vi "OE2031&OE2041_DATA Transmit.vi"(0 "Input Data":u8[](array[numeric]), 1 "Remote Mode":u16(ring) items=["USB"=0, "Ethernet"=3]) -> (2 "Total Data Array":dbl[][](array[numeric]), 3 "Parameter Values":T2, 4 "Trig_Count":u8[](array[numeric]), 5 "PLL&Overload":T1)   [LabVIEW 2011]
panel:
  out "Group":u16
  out "X":dbl[](array[numeric])
  out "Y":dbl[](array[numeric])
  out "Frequency":dbl[](array[numeric])
  out "XNoise":dbl[](array[numeric])
  out "XD1":dbl[](array[numeric])
  out "YD1":dbl[](array[numeric])
  out "XD2":dbl[](array[numeric])
  out "YD2":dbl[](array[numeric])
  out "AUXADC1":dbl[](array[numeric])
  out "AUXADC2":dbl[](array[numeric])
  out "AUXADC3":dbl[](array[numeric])
  out "AUXADC4":dbl[](array[numeric])
  out "XD3":dbl[](array[numeric])
  out "YD3":dbl[](array[numeric])
  out "YNoise":dbl[](array[numeric])
  out "R":dbl[](array[numeric])
  out "Xita":dbl[](array[numeric])
  out "RD1":dbl[](array[numeric])
  out "XitaD1":dbl[](array[numeric])
  out "RD2":dbl[](array[numeric])
  out "XitaD2":dbl[](array[numeric])
  out "RD3":dbl[](array[numeric])
  out "XitaD3":dbl[](array[numeric])
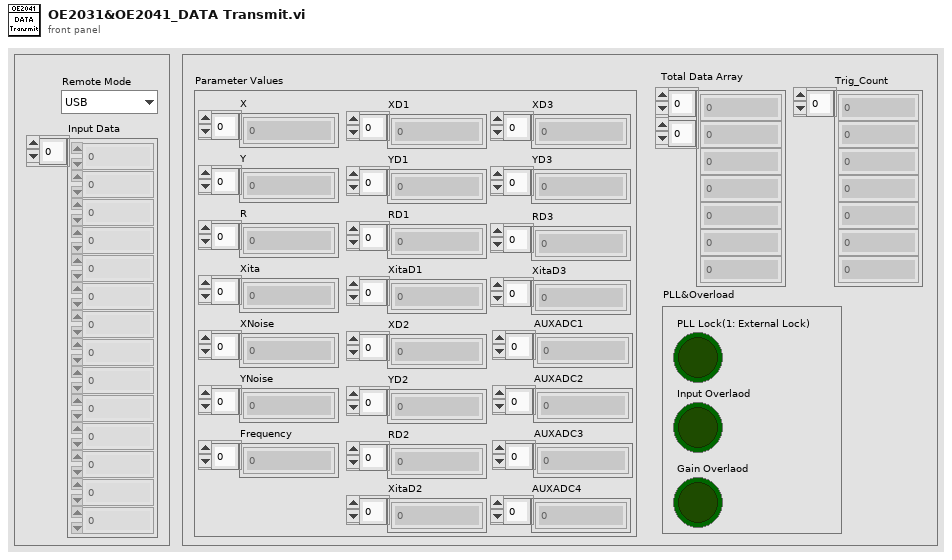
[diagram p1: front panel]
types:
  T1 = cluster{"PLL Lock(1: External Lock)":bool, "Input Overlaod":bool, "Gain Overlaod":bool}
  T2 = cluster{"X":dbl[], "Y":dbl[], "R":dbl[], "Xita":dbl[], "XNoise":dbl[], "YNoise":dbl[], "Frequency":dbl[], "XD1":dbl[], "YD1":dbl[], "RD1":dbl[], "XitaD1":dbl[], "XD2":dbl[], "YD2":dbl[], "RD2":dbl[], "XitaD2":dbl[], "XD3":dbl[], "YD3":dbl[], "RD3":dbl[], "XitaD3":dbl[], "AUXADC1":dbl[], "AUXADC2":dbl[], "AUXADC3":dbl[], "AUXADC4":dbl[]}
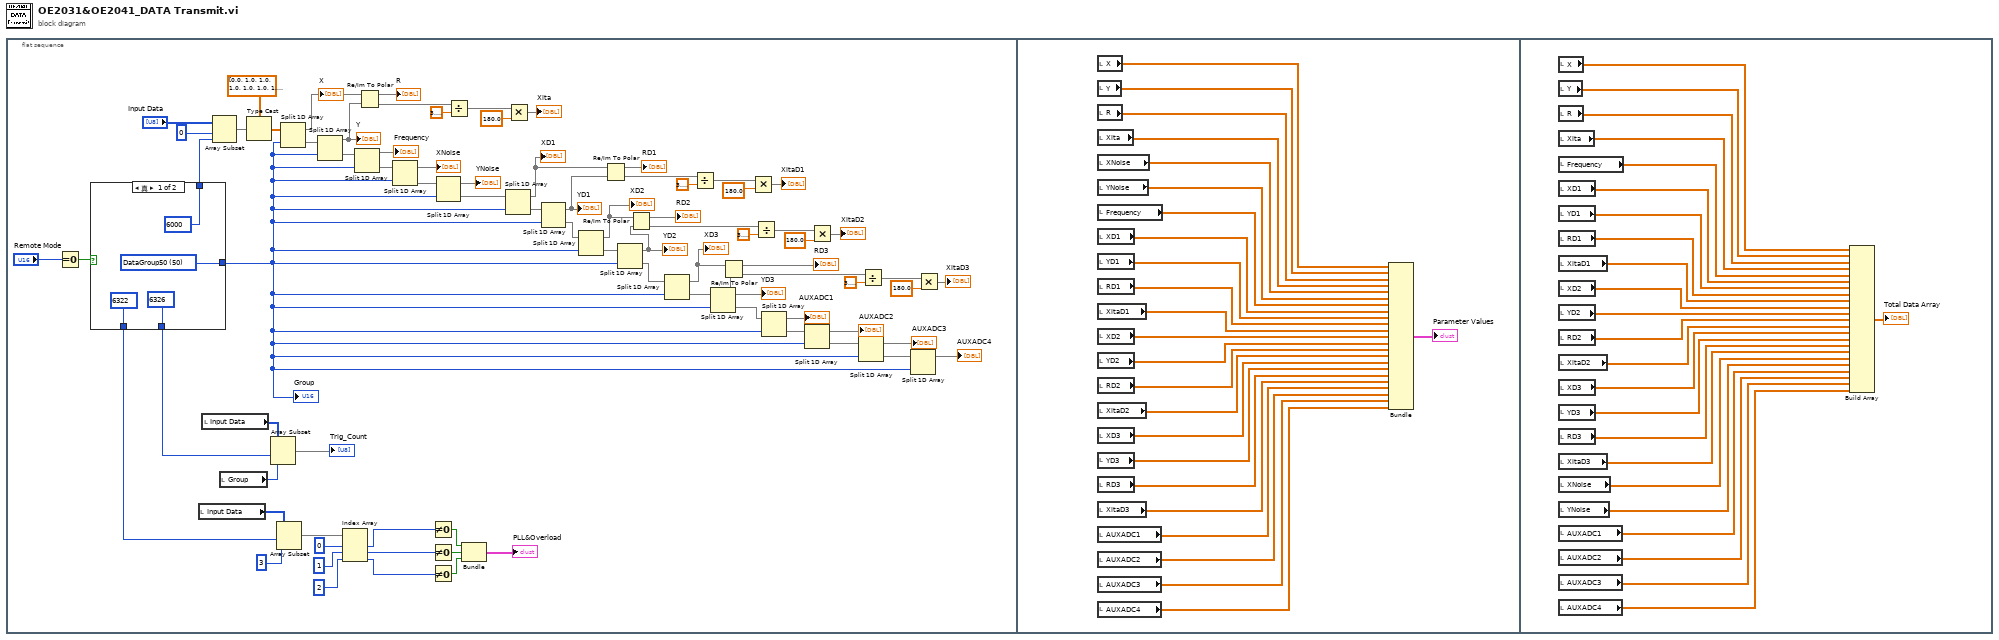
[diagram p0: block diagram]
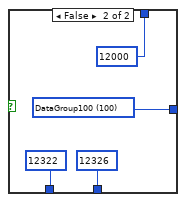
[diagram p2: hidden frame]
diagram:
  n1 = flat-sequence {
    frame #0 {
      n2 = Equal To 0?(x="Remote Mode") -> (x = 0?=w18:bool)
      n3 = case shown="真" w18 {
        tunnel: [w84 w88] -> w20
        tunnel: [6000 ("长度") 12000 ("长度")] -> w23
        tunnel: [6326 ("索引") 12326 ("索引")] -> w16
        tunnel: [6322 ("索引") 12322 ("索引")] -> w1
        frame True {
          w84 = u16 50 items=["unsignedInt8"=1, "unsignedInt16"=2, "unsignedInt32"=4, "unsignedInt64"=8, "Float"=80, "Double"=160, "StartLength"=2240, "DataGroup50"=50, "DataGroup100"=100, "DataGroup20"=20] ("数据类型")
        }
        frame False {
          w88 = u16 100 items=["unsignedInt8"=1, "unsignedInt16"=2, "unsignedInt32"=4, "unsignedInt64"=8, "Float"=80, "Double"=160, "StartLength"=2240, "DataGroup50"=50, "DataGroup100"=100, "DataGroup20"=20] ("数据类型")
        }
      }
      "Group" <- w20
      n4 = local read "Input Data"() -> (w14:u8[])
      n5 = local read "Input Data"() -> (w22:u8[])
      n6 = Array Subset(array="Input Data", index=0 ("索引"), length=w23) -> (w77:u8[])
      n7 = local read "Group"() -> (w19:u16)
      n8 = Type Cast(type=dbl[] [0.0, 1.0, 1.0, 1.0, 1.0, 1.0, 1.0, 1.0, 1.0, 1.0, 1.0, 1.0, 1.0, 1.0, 1.0, 1.0, 1.0, 1.0, 1.0, 1.0, 1.0, 1.0, 1.0, 1.0, 1.0, 1.0, 1.0, 1.0, 1.0, 1.0, 1.0, 1.0, 1.0, 1.0, 1.0, 1.0, 1.0, 1.0, 1.0, 1.0, 1.0, 1.0, 1.0, 1.0, 1.0, 1.0, 1.0, 1.0, 1.0, 1.0, 1.0, 1.0, 1.0, 1.0, 1.0, 1.0, 1.0, 1.0, 1.0, 1.0, 1.0, 1.0, 1.0, 1.0, 1.0, 1.0, 1.0, 1.0, 1.0, 1.0, 1.0, 1.0, 1.0, 1.0, 1.0, 1.0, 1.0, 1.0, 1.0, 1.0, 1.0, 1.0, 1.0, 1.0, 1.0, 1.0, 1.0, 1.0, 1.0, 1.0, 1.0, 1.0, 1.0, 1.0, 1.0, 1.0, 1.0, 1.0, 1.0, 1.0, 1.0, 1.0, 1.0, 1.0, 1.0, 1.0, 1.0, 1.0, 1.0, 1.0, 1.0, 1.0, 1.0, 1.0, 1.0, 1.0, 1.0, 1.0, 1.0, 1.0, 1.0, 1.0, 1.0, 1.0, 1.0, 1.0, 1.0, 1.0, 1.0, 1.0, 1.0, 1.0, 1.0, 1.0, 1.0, 1.0, 1.0, 1.0, 1.0, 1.0, 1.0, 1.0, 1.0, 1.0, 1.0, 1.0, 1.0, 1.0, 1.0, 1.0, 1.0, 1.0, 1.0, 1.0, 1.0, 1.0, 1.0, 1.0, 1.0, 1.0, 1.0, 1.0, 1.0, 1.0, 1.0, 1.0, 1.0, 1.0, 1.0, 1.0, 1.0, 1.0, 1.0, 1.0, 1.0, 1.0, 1.0, 1.0, 1.0, 1.0, 1.0, 1.0, 1.0, 1.0, 1.0, 1.0, 1.0, 1.0, 1.0, 1.0, 1.0, 1.0, 1.0, 1.0, 1.0, 1.0, 1.0, 1.0, 1.0, 1.0, 1.0, 1.0, 1.0, 1.0, 1.0, 1.0, 1.0, 1.0, 1.0, 1.0, 1.0, 1.0, 1.0, 1.0, 1.0, 1.0, 1.0, 1.0, 1.0, 1.0, 1.0, 1.0, 1.0, 1.0, 1.0, 1.0, 1.0, 1.0, 1.0, 1.0, 1.0, 1.0, 1.0, 1.0, 1.0, 1.0, 1.0, 1.0, 1.0, 1.0, 1.0, 1.0, 1.0, 1.0, 1.0, 1.0, 1.0, 1.0, 1.0, 1.0, 1.0, 1.0, 1.0, 1.0, 1.0, 1.0, 1.0, 1.0, 1.0, 1.0, 1.0, 1.0, 1.0, 1.0, 1.0, 1.0, 1.0, 1.0, 1.0, 1.0, 1.0, 1.0, 1.0, 1.0, 1.0, 1.0, 1.0, 1.0, 1.0, 1.0, 1.0, 1.0, 1.0, 1.0, 1.0, 1.0, 1.0, 1.0, 1.0, 1.0, 1.0, 1.0, 1.0, 1.0, 1.0, 1.0, 1.0, 1.0, 1.0, 1.0, 1.0, 1.0, 1.0, 1.0, 1.0, 1.0, 1.0, 1.0, 1.0, 1.0, 1.0, 1.0, 1.0, 1.0, 1.0, 1.0, 1.0, 1.0, 1.0, 1.0, 1.0, 1.0, 1.0, 1.0, 1.0, 1.0, 1.0, 1.0, 1.0, 1.0, 1.0, 1.0, 1.0, 1.0, 1.0, 1.0, 1.0, 1.0, 1.0, 1.0, 1.0, 1.0, 1.0, 1.0, 1.0, 1.0, 1.0, 1.0, 1.0, 1.0, 1.0, 1.0, 1.0, 1.0, 1.0, 1.0, 1.0, 1.0, 1.0, 1.0, 1.0, 1.0, 1.0, 1.0, 1.0, 1.0, 1.0, 1.0, 1.0, 1.0, 1.0, 1.0, 1.0, 1.0, 1.0, 1.0, 1.0, 1.0, 1.0, 1.0, 1.0, 1.0, 1.0, 1.0, 1.0, 1.0, 1.0, 1.0, 1.0, 1.0, 1.0, 1.0, 1.0, 1.0, 1.0, 1.0, 1.0, 1.0, 1.0, 1.0, 0.0, 1.0, 1.0, 1.0, 1.0, 1.0, 1.0, 1.0, 1.0, 1.0, 1.0, 1.0, 1.0, 1.0, 1.0, 1.0, 1.0, 1.0, 1.0, 1.0, 1.0, 1.0, 1.0, 1.0, 1.0, 1.0, 1.0, 1.0, 1.0, 1.0, 1.0, 1.0, 1.0, 1.0, 1.0, 1.0, 1.0, 1.0, 1.0, 1.0, 1.0, 1.0, 1.0, 1.0, 1.0, 1.0, 1.0, 1.0, 1.0, 1.0, 1.0, 1.0, 1.0, 1.0, 1.0, 1.0, 1.0, 1.0, 1.0, 1.0, 1.0, 1.0, 1.0, 1.0, 1.0, 1.0, 1.0, 1.0, 1.0, 1.0, 1.0, 1.0, 1.0, 1.0, 1.0, 1.0, 1.0, 1.0, 1.0, 1.0, 1.0, 1.0, 1.0, 1.0, 1.0, 1.0, 1.0, 1.0, 1.0, 1.0, 1.0, 1.0, 1.0, 1.0, 1.0, 1.0, 1.0, 1.0, 1.0, 1.0, 1.0, 1.0, 1.0, 1.0, 1.0, 1.0, 1.0, 1.0, 1.0, 1.0, 1.0, 1.0, 1.0, 1.0, 1.0, 1.0, 1.0, 1.0, 1.0, 1.0, 1.0, 1.0, 1.0, 1.0, 1.0, 1.0, 1.0, 1.0, 1.0, 1.0, 1.0, 1.0, 1.0, 1.0, 1.0, 1.0, 1.0, 1.0, 1.0, 1.0, 1.0, 1.0, 1.0, 1.0, 1.0, 1.0, 1.0, 1.0, 1.0, 1.0, 1.0, 1.0, 1.0, 1.0, 1.0, 1.0, 1.0, 1.0, 1.0, 1.0, 1.0, 1.0, 1.0, 1.0, 1.0, 1.0, 1.0, 1.0, 1.0, 1.0, 1.0, 1.0, 1.0, 1.0, 1.0, 1.0, 1.0, 1.0, 1.0, 1.0, 1.0, 1.0, 1.0, 1.0, 1.0, 1.0, 1.0, 1.0, 1.0, 1.0, 1.0, 1.0, 1.0, 1.0, 1.0, 1.0, 1.0, 1.0, 1.0, 1.0, 1.0, 1.0, 1.0, 1.0, 1.0, 1.0, 1.0, 1.0, 1.0, 1.0, 1.0, 1.0, 1.0, 1.0, 1.0, 1.0, 1.0, 1.0, 1.0, 1.0, 1.0, 1.0, 1.0, 1.0, 1.0, 1.0, 1.0, 1.0, 1.0, 1.0, 1.0, 1.0, 1.0, 1.0, 1.0, 1.0, 1.0, 1.0, 1.0, 1.0, 1.0, 1.0, 1.0, 1.0, 1.0, 1.0, 1.0, 1.0, 1.0, 1.0, 1.0, 1.0, 1.0, 1.0, 1.0, 1.0, 1.0, 1.0, 1.0, 1.0, 1.0, 1.0, 1.0, 1.0, 1.0, 1.0, 1.0, 1.0, 1.0, 1.0, 1.0, 1.0, 1.0, 1.0, 1.0, 1.0, 1.0, 1.0, 1.0, 1.0, 1.0, 1.0, 1.0, 1.0, 1.0, 1.0, 1.0, 1.0, 1.0, 1.0, 1.0, 1.0, 1.0, 1.0, 1.0, 1.0, 1.0, 1.0, 1.0, 1.0, 1.0, 1.0, 1.0, 1.0, 1.0, 1.0, 1.0, 1.0, 1.0, 1.0, 1.0, 1.0, 1.0, 1.0, 1.0, 1.0, 1.0, 1.0, 1.0, 1.0, 1.0, 1.0, 1.0, 1.0, 1.0, 1.0, 1.0, 1.0, 1.0, 1.0, 1.0, 1.0, 1.0, 1.0, 1.0, 1.0, 1.0, 1.0, 1.0, 1.0, 1.0, 1.0, 1.0, 1.0, 1.0, 1.0, 1.0, 1.0, 1.0, 1.0, 1.0, 1.0, 1.0, 1.0, 1.0, 1.0, 1.0, 1.0, 1.0, 1.0, 1.0, 1.0, 1.0, 1.0, 1.0, 1.0, 1.0, 1.0, 1.0, 1.0, 1.0, 1.0, 1.0, 1.0, 1.0, 1.0, 1.0, 1.0, 1.0, 1.0, 1.0, 1.0, 1.0, 1.0, 1.0, 1.0, 1.0, 1.0, 1.0, 1.0, 1.0, 1.0, 1.0, 1.0, 1.0, 1.0, 1.0, 1.0, 1.0, 1.0], x=w77) -> (*(type *) &x=w65:dbl[])
      n9 = Array Subset(array=w22, index=w16, length=w19) -> (→"Trig_Count":u8[])
      n10 = Array Subset(array=w14, index=w1, length=3 ("长度")) -> (w12:u8[])
      n11 = Split 1D Array(array=w65, index=w20) -> (first subarray=w52:dbl[], second subarray=w66:dbl[])
      "X" <- w52
      n12 = Split 1D Array(array=w66, index=w20) -> (first subarray=w51:dbl[], second subarray=w78:dbl[])
      "Y" <- w51
      n13 = Index Array(array=w12, index #1=0 ("索引"), index #2=1 ("索引"), index #3=2 ("索引")) -> (element #1=w4:u8, element #2=w3:u8, element #3=w2:u8)
      n14 = Split 1D Array(array=w78, index=w20) -> (first subarray=→"Frequency":dbl[], second subarray=w56:dbl[])
      n15 = Re/Im To Polar(2:w51, 3:w52) -> (0:w50:dbl[], 1:→"R":dbl[])
      n16 = Split 1D Array(array=w56, index=w20) -> (first subarray=→"XNoise":dbl[], second subarray=w58:dbl[])
      n17 = Not Equal To 0?(x=w4) -> (x != 0?=w7:bool)
      n18 = Not Equal To 0?(x=w3) -> (x != 0?=w8:bool)
      n19 = Not Equal To 0?(x=w2) -> (x != 0?=w6:bool)
      n20 = Split 1D Array(array=w58, index=w20) -> (first subarray=→"YNoise":dbl[], second subarray=w57:dbl[])
      n21 = Divide(x=w50, y=3.141592653589793) -> (x/y=w54:dbl[])
      n22 = Bundle(w7, w8, w6) -> (→"PLL&Overload":cluster{bool, bool, bool})  [unwired: 1 in]
      n23 = Split 1D Array(array=w57, index=w20) -> (first subarray=w29:dbl[], second subarray=w69:dbl[])
      "XD1" <- w29
      n24 = Multiply(x=w54, y=180.0) -> (x*y=→"Xita":dbl[])
      n25 = Split 1D Array(array=w69, index=w20) -> (first subarray=w28:dbl[], second subarray=w79:dbl[])
      "YD1" <- w28
      n26 = Split 1D Array(array=w79, index=w20) -> (first subarray=w27:dbl[], second subarray=w80:dbl[])
      "XD2" <- w27
      n27 = Re/Im To Polar(2:w28, 3:w29) -> (0:w45:dbl[], 1:→"RD1":dbl[])
      n28 = Split 1D Array(array=w80, index=w20) -> (first subarray=w26:dbl[], second subarray=w60:dbl[])
      "YD2" <- w26
      n29 = Re/Im To Polar(2:w26, 3:w27) -> (0:w38:dbl[], 1:→"RD2":dbl[])
      n30 = Split 1D Array(array=w60, index=w20) -> (first subarray=w25:dbl[], second subarray=w62:dbl[])
      "XD3" <- w25
      n31 = Divide(x=w45, y=3.141592653589793) -> (x/y=w43:dbl[])
      n32 = Split 1D Array(array=w62, index=w20) -> (first subarray=w24:dbl[], second subarray=w61:dbl[])
      "YD3" <- w24
      n33 = Re/Im To Polar(2:w24, 3:w25) -> (0:w33:dbl[], 1:→"RD3":dbl[])
      n34 = Multiply(x=w43, y=180.0) -> (x*y=→"XitaD1":dbl[])
      n35 = Divide(x=w38, y=3.141592653589793) -> (x/y=w40:dbl[])
      n36 = Split 1D Array(array=w61, index=w20) -> (first subarray=→"AUXADC1":dbl[], second subarray=w70:dbl[])
      n37 = Split 1D Array(array=w70, index=w20) -> (first subarray=→"AUXADC2":dbl[], second subarray=w76:dbl[])
      n38 = Multiply(x=w40, y=180.0) -> (x*y=→"XitaD2":dbl[])
      n39 = Split 1D Array(array=w76, index=w20) -> (first subarray=→"AUXADC3":dbl[], second subarray=w75:dbl[])
      n40 = Divide(x=w33, y=3.141592653589793) -> (x/y=w31:dbl[])
      n41 = Split 1D Array(array=w75, index=w20) -> (first subarray=→"AUXADC4":dbl[])  [unwired: 1 out]
      n42 = Multiply(x=w31, y=180.0) -> (x*y=→"XitaD3":dbl[])
    }
    frame #1 {
      n43 = local read "X"() -> (w112:dbl[])
      n44 = local read "Y"() -> (w111:dbl[])
      n45 = local read "R"() -> (w110:dbl[])
      n46 = local read "Xita"() -> (w109:dbl[])
      n47 = local read "XNoise"() -> (w108:dbl[])
      n48 = local read "YNoise"() -> (w107:dbl[])
      n49 = local read "Frequency"() -> (w106:dbl[])
      n50 = local read "XD1"() -> (w101:dbl[])
      n51 = local read "YD1"() -> (w100:dbl[])
      n52 = local read "RD1"() -> (w99:dbl[])
      n53 = local read "XitaD1"() -> (w98:dbl[])
      n54 = local read "XD2"() -> (w97:dbl[])
      n55 = local read "YD2"() -> (w96:dbl[])
      n56 = local read "RD2"() -> (w95:dbl[])
      n57 = local read "XitaD2"() -> (w94:dbl[])
      n58 = local read "XD3"() -> (w93:dbl[])
      n59 = local read "YD3"() -> (w92:dbl[])
      n60 = local read "RD3"() -> (w91:dbl[])
      n61 = local read "XitaD3"() -> (w90:dbl[])
      n62 = local read "AUXADC1"() -> (w102:dbl[])
      n63 = local read "AUXADC2"() -> (w103:dbl[])
      n64 = local read "AUXADC3"() -> (w104:dbl[])
      n65 = local read "AUXADC4"() -> (w105:dbl[])
      n66 = Bundle("X"=w112, "Y"=w111, "R"=w110, "Xita"=w109, "XNoise"=w108, "YNoise"=w107, "Frequency"=w106, "XD1"=w101, "YD1"=w100, "RD1"=w99, "XitaD1"=w98, "XD2"=w97, "YD2"=w96, "RD2"=w95, "XitaD2"=w94, "XD3"=w93, "YD3"=w92, "RD3"=w91, "XitaD3"=w90, "AUXADC1"=w102, "AUXADC2"=w103, "AUXADC3"=w104, "AUXADC4"=w105) -> (→"Parameter Values":T2)  [unwired: 1 in]
    }
    frame #2 {
      n67 = local read "X"() -> (w116:dbl[])
      n68 = local read "Y"() -> (w117:dbl[])
      n69 = local read "R"() -> (w118:dbl[])
      n70 = local read "Xita"() -> (w119:dbl[])
      n71 = local read "Frequency"() -> (w120:dbl[])
      n72 = local read "XD1"() -> (w125:dbl[])
      n73 = local read "YD1"() -> (w126:dbl[])
      n74 = local read "RD1"() -> (w127:dbl[])
      n75 = local read "XitaD1"() -> (w128:dbl[])
      n76 = local read "XD2"() -> (w129:dbl[])
      n77 = local read "YD2"() -> (w130:dbl[])
      n78 = local read "RD2"() -> (w131:dbl[])
      n79 = local read "XitaD2"() -> (w132:dbl[])
      n80 = local read "XD3"() -> (w133:dbl[])
      n81 = local read "YD3"() -> (w134:dbl[])
      n82 = local read "RD3"() -> (w135:dbl[])
      n83 = local read "XitaD3"() -> (w136:dbl[])
      n84 = local read "XNoise"() -> (w113:dbl[])
      n85 = local read "YNoise"() -> (w114:dbl[])
      n86 = local read "AUXADC1"() -> (w124:dbl[])
      n87 = local read "AUXADC2"() -> (w123:dbl[])
      n88 = local read "AUXADC3"() -> (w122:dbl[])
      n89 = local read "AUXADC4"() -> (w121:dbl[])
      n90 = Build Array(w116, w117, w118, w119, w120, w125, w126, w127, w128, w129, w130, w131, w132, w133, w134, w135, w136, w113, w114, w124, w123, w122, w121) -> (→"Total Data Array":dbl[][])
    }
  }
